vi "Optics.vi"   [LabVIEW 2021]
types:
  T1 = enum16{"_Quit_", "Init", "Ready", "CCD_shot", "QueueData", "HTL", "BG_Setup", "Error Handler"}
  T2 = enum16{"BGShot", "SequenceShot", "SingleShot", "default"}
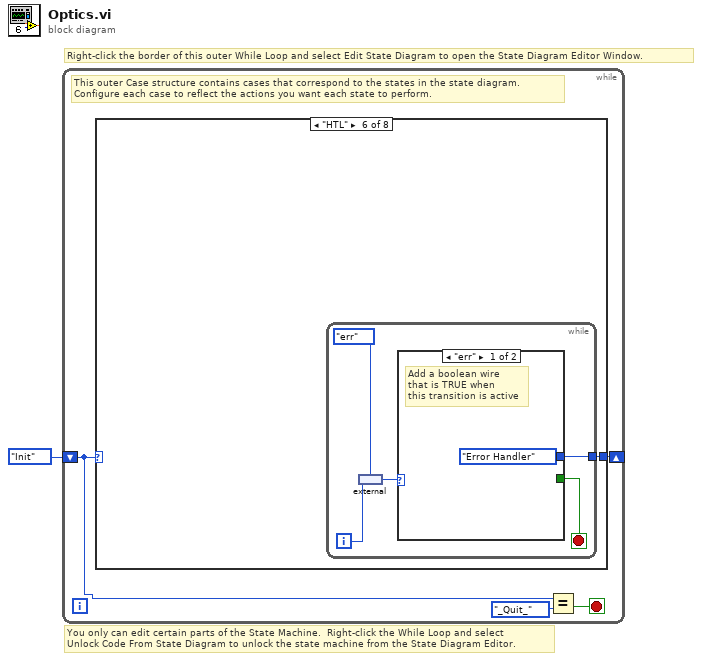
[diagram p0: block diagram]
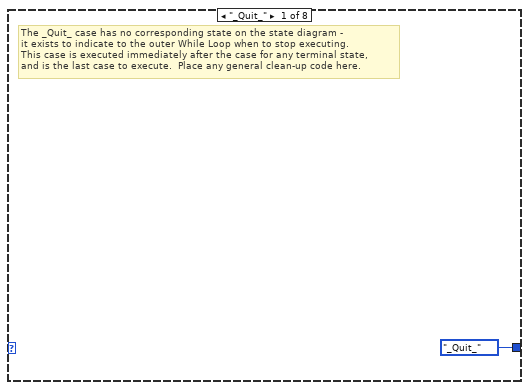
[diagram p2: hidden frame]
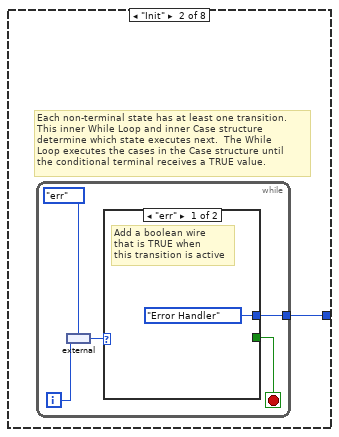
[diagram p3: hidden frame]
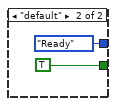
[diagram p4: hidden frame]
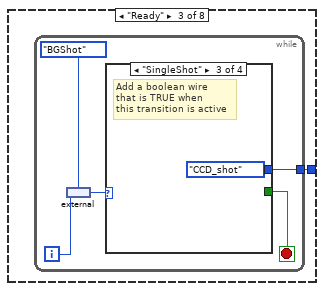
[diagram p5: hidden frame]
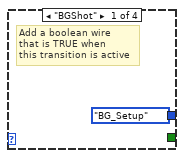
[diagram p6: hidden frame]
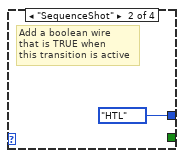
[diagram p7: hidden frame]
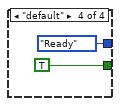
[diagram p8: hidden frame]
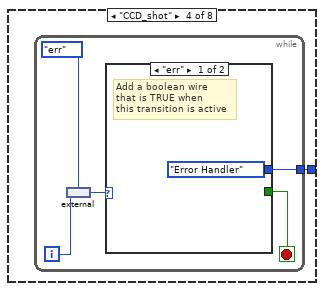
[diagram p9: hidden frame]
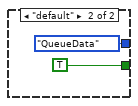
[diagram p10: hidden frame]
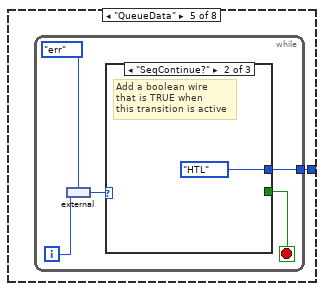
[diagram p11: hidden frame]
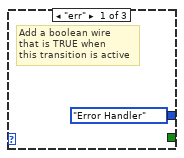
[diagram p12: hidden frame]
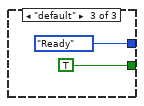
[diagram p13: hidden frame]
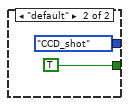
[diagram p14: hidden frame]
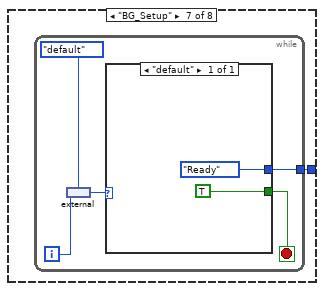
[diagram p15: hidden frame]
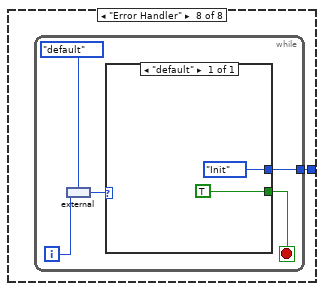
[diagram p16: hidden frame]
diagram:
  # "Right-click the border of this outer While Loop and select Edit State Diagram to open the State Diagram Editor Window."
  # "You only can edit certain parts of the State Machine.  Right-click the While Loop and select \nUnlock Code From State Diagram to unlock the state machine from the State Diagram Editor."
  n1 = while {
    shift-right: [w4] -> _
    shift-left: T1."Init" -> [w5]
    stop <- w3 stop-if-true
    # "This outer Case structure contains cases that correspond to the states in the state diagram.  \nConfigure each case to reflect the actions you want each state to perform."
    n2 = case shown="\"HTL\"" w5 {
      tunnel: [T1."_Quit_" w7 w21 w37 w51 w66 w80 w93] -> w4
      frame "_Quit_" {
        # "The _Quit_ case has no corresponding state on the state diagram -\nit exists to indicate to the outer While Loop when to stop executing.\nThis case is executed immediately after the case for any terminal state, \nand is the last case to execute.  Place any general clean-up code here."
      }
      frame "Init" {
        # "Each non-terminal state has at least one transition.\nThis inner While Loop and inner Case structure \ndetermine which state executes next.  The While \nLoop executes the cases in the Case structure until \nthe conditional terminal receives a TRUE value."
        n3 = while {
          tunnel: [w9] -> w7
          i -> [w12]
          stop <- w8 stop-if-true
          n4 = external(enum16{"err", "default"}."err", w12) -> (w10:enum16{"err", "default"})
          n5 = case shown="\"err\"" w10 {
            tunnel: [T1."Error Handler" T1."Ready"] -> w9
            tunnel: [_ TRUE] -> w8
            frame "err" {
              # "Add a boolean wire\nthat is TRUE when\nthis transition is active"
            }
            frame "default" {
            }
          }
        }
      }
      frame "Ready" {
        n6 = while {
          tunnel: [w23] -> w21
          i -> [w26]
          stop <- w22 stop-if-true
          n7 = external(T2."BGShot", w26) -> (w24:T2)
          n8 = case shown="\"SingleShot\"" w24 {
            tunnel: [T1."BG_Setup" T1."HTL" T1."CCD_shot" T1."Ready"] -> w23
            tunnel: [_ _ _ TRUE] -> w22
            frame "BGShot" {
              # "Add a boolean wire\nthat is TRUE when\nthis transition is active"
            }
            frame "SequenceShot" {
              # "Add a boolean wire\nthat is TRUE when\nthis transition is active"
            }
            frame "SingleShot" {
              # "Add a boolean wire\nthat is TRUE when\nthis transition is active"
            }
            frame "default" {
            }
          }
        }
      }
      frame "CCD_shot" {
        n9 = while {
          tunnel: [w39] -> w37
          i -> [w42]
          stop <- w38 stop-if-true
          n10 = external(enum16{"err", "default"}."err", w42) -> (w40:enum16{"err", "default"})
          n11 = case shown="\"err\"" w40 {
            tunnel: [T1."Error Handler" T1."QueueData"] -> w39
            tunnel: [_ TRUE] -> w38
            frame "err" {
              # "Add a boolean wire\nthat is TRUE when\nthis transition is active"
            }
            frame "default" {
            }
          }
        }
      }
      frame "QueueData" {
        n12 = while {
          tunnel: [w53] -> w51
          i -> [w56]
          stop <- w52 stop-if-true
          n13 = external(enum16{"err", "SeqContinue?", "default"}."err", w56) -> (w54:enum16{"err", "SeqContinue?", "default"})
          n14 = case shown="\"SeqContinue?\"" w54 {
            tunnel: [T1."Error Handler" T1."HTL" T1."Ready"] -> w53
            tunnel: [_ _ TRUE] -> w52
            frame "err" {
              # "Add a boolean wire\nthat is TRUE when\nthis transition is active"
            }
            frame "SeqContinue?" {
              # "Add a boolean wire\nthat is TRUE when\nthis transition is active"
            }
            frame "default" {
            }
          }
        }
      }
      frame "HTL" {
        n15 = while {
          tunnel: [w68] -> w66
          i -> [w71]
          stop <- w67 stop-if-true
          n16 = external(enum16{"err", "default"}."err", w71) -> (w69:enum16{"err", "default"})
          n17 = case shown="\"err\"" w69 {
            tunnel: [T1."Error Handler" T1."CCD_shot"] -> w68
            tunnel: [_ TRUE] -> w67
            frame "err" {
              # "Add a boolean wire\nthat is TRUE when\nthis transition is active"
            }
            frame "default" {
            }
          }
        }
      }
      frame "BG_Setup" {
        n18 = while {
          tunnel: [w82] -> w80
          i -> [w85]
          stop <- w81 stop-if-true
          n19 = external(enum16{"default"}."default", w85) -> (w83:enum16{"default"})
          n20 = case shown="\"default\"" w83 {
            tunnel: [T1."Ready"] -> w82
            tunnel: [TRUE] -> w81
            frame "default" {
            }
          }
        }
      }
      frame "Error Handler" {
        n21 = while {
          tunnel: [w95] -> w93
          i -> [w98]
          stop <- w94 stop-if-true
          n22 = external(enum16{"default"}."default", w98) -> (w96:enum16{"default"})
          n23 = case shown="\"default\"" w96 {
            tunnel: [T1."Init"] -> w95
            tunnel: [TRUE] -> w94
            frame "default" {
            }
          }
        }
      }
    }
    n24 = Equal?(x=w5, y=T1."_Quit_") -> (x = y?=w3:bool)
  }
